vi "SCCAPI Find All Providers.vi"(8 "error in (no error)":errorcluster, 11 "provider location":string) -> (0 "error out":errorcluster, 1 "additional information":string[](array[string]), 2 "providers location":string[](array[string]), 3 "provider names":string[](array[string]))   [LabVIEW 2017, in "NI_SCC.lvlib"]
uses:
  <vilib>/SourceControl/sccapi/NI_SCC.lvlib
  <vilib>/SourceControl/sccapi/SCCAPI SCC Operations.ctl
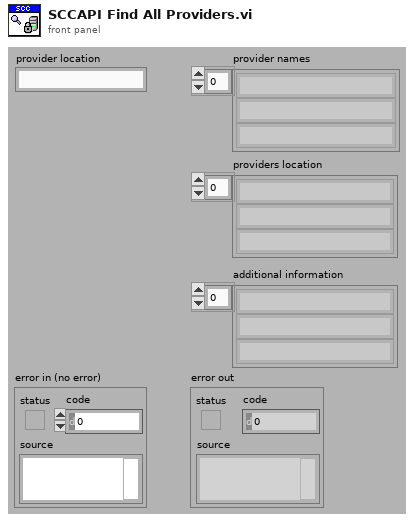
[diagram p1: front panel]
types:
  T1 = typedef "NI_SCC.lvlib/SCCAPI SCC Operations.ctl" = enum16{"Add", "Check In", "Check Out", "Close Project", "Compare Files", "Compare VIs", "Configure Project", "File History", "File Properties", "File Status", "Find All Providers", "Get Advanced Command Options", "Get File Copy", "Get Latest Version", "Get Project Name", "Get StaticVI Path", "Initialize", "Not A Source Control Reference", "Open Project", "Provider Supports Functionality", "Remove", "Run Provider", "Undo Check Out", "Uninitialize", "Is File In Local Path"}
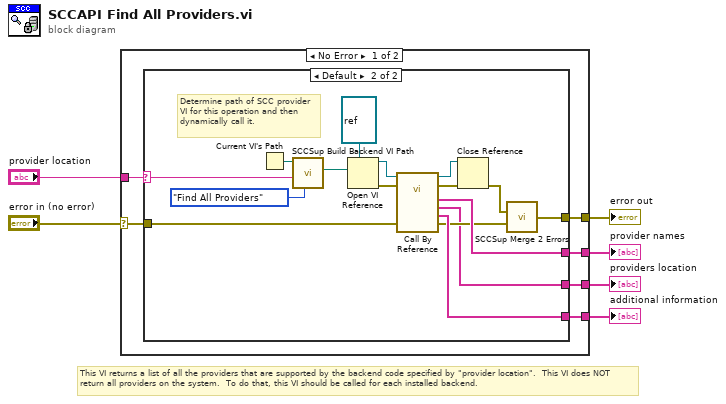
[diagram p0: block diagram]
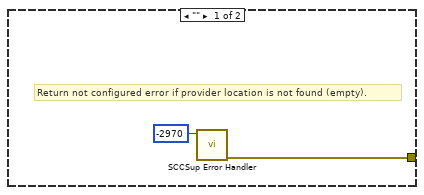
[diagram p2: hidden frame]
diagram:
  # "This VI returns a list of all the providers that are supported by the backend code specified by \"provider location\".  This VI does NOT return all providers on the system.  To do that, this VI should be called for each installed backend."
  n1 = case shown="No Error" "error in (no error)" {
    selector: "error in (no error)" -> [w7 w31]
    tunnel: [w12 w31] -> w5
    tunnel: [w11 _] -> w4
    tunnel: [w10 _] -> w3
    tunnel: [w9 _] -> w2
    tunnel: "provider location" -> [w8 _]
    frame No Error {
      n2 = case shown="Default" w8 {
        selector: w8 -> [_ w16]
        tunnel: [w13 w30] -> w12
        tunnel: [_ w24] -> w11
        tunnel: [_ w23] -> w10
        tunnel: [_ w17] -> w9
        tunnel: w7 -> [_ w15]
        frame "" {
          # "Return not configured error if provider location is not found (empty)."
          n3 = call <vilib>:"SCCSup Error Handler.vi"("scc error code"=-2970 ("code")) -> ("error out"=w13:errorcluster)  [unwired: 10 in]
        }
        frame Default {
          # "Determine path of SCC provider VI for this operation and then dynamically call it."
          n4 = Current VI's Path() -> (path=w20:path)
          n5 = call <vilib>:"SCCSup Build Backend VI Path.vi"("scc operation"=SCCAPI_SCC_Operations."Find All Providers", "provider location"=w16, "caller path"=w20) -> ("scc backend VI path"=w18:path)  [unwired: 8 in]
          n6 = Open VI Reference(type specifier VI Refnum (for type only)=refnum<vi> refnum, vi path=w18) -> (vi reference=w28:refnum<vi>, error out=w27:errorcluster)  [unwired: 4 in]
          n7 = call-by-ref "?"(reference=w28, error in=w27, "error in (no error)"=w15) -> (reference out=w26:refnum<vi>, error out=w25:errorcluster, 0:"error out"=w21:errorcluster, "additional data"=w23:string[], "provider locations"=w17:string[], "provider names"=w24:string[])  [unwired: 7 in]
          n8 = Close Reference(reference=w26, error in (no error)=w25) -> (error out=w22:errorcluster)
          n9 = call <vilib>:"SCCSup Merge 2 Errors.vi"("Error IO 1"=w22, "Error IO 2"=w21) -> ("Error IO out"=w30:errorcluster)  [unwired: 13 in]
        }
      }
    }
    frame Error {
    }
  }
  "error out" <- w5
  "provider names" <- w4
  "additional information" <- w3
  "providers location" <- w2
